vi "Vision Shooter Auto Target.vi"(11 "navX Device":T1={"Interface"={"Protocol"=enum."SERIAL", "Update Rate (4Hz-60Hz)"=4, "navX Open TypeDef"=variant}, "Notify Packet"=refnum, "Loop VI Refnum"=refnum, "Ready to Close Occurrence Refnum"=refnum} {"Interface"."Update Rate (4Hz-60Hz)" min=4 max=60 step=1}) -> ()   [LabVIEW 2015]
uses:
  NavX/navX Library v2/TypeDefs/Z900_navX_DeviceTypeDef.ctl
  NavX/navX Library v2/TypeDefs/Z900_navX_ProtocolTypeDef.ctl
  NavX/navX Library v2/TypeDefs/Z900_navX_NotifyPacketTypeDef.ctl
  NavX/navX Library v2/TypeDefs/Z900_navX_ActionTypeDef.ctl
  Team Code/Robot Global Data.vi
  <vilib>/Rock Robotics/Network Tables/NT Write Number.vi
  NavX/navX Library v2/navX Library v2.lvlib
panel:
  in  "Vertical Linear Relationship":dbl
  out "VisionVertical":cluster{"VisionGyroTarget":dbl, dbl, dbl}(graph)
  out "VisionStateDistance":enum16{"Disabled", "Enable", "Suspended", "PID"}(ring)
  in  "VeriticalOffset":dbl=0.033
  in  "X Gain":dbl=80.0
  in  "minimumVisionValue":dbl=0.45
  out "VisionHorizontal":cluster{"VisionGyroTarget":dbl, dbl, dbl}(graph)
  out "VisionStateAngle":enum16{"Disabled", "Enable", "Suspended", "PID"}(ring)
  in  "HorizontalOffset":dbl=0.066
  # "More positive = counter clockwise\nMore negative = clockwise"
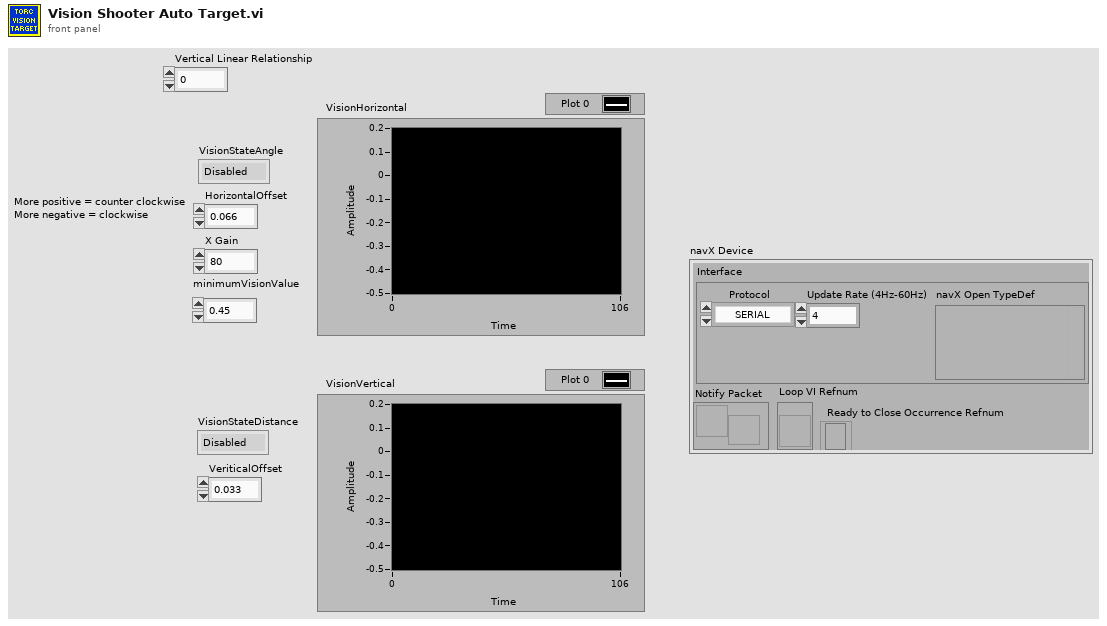
[diagram p1: front panel]
types:
  T1 = typedef "navX Library v2.lvlib/Z900_navX_DeviceTypeDef.ctl" = cluster{"Interface":cluster{"Protocol":T2, "Update Rate (4Hz-60Hz)":u8, "navX Open TypeDef":variant}, "Notify Packet":refnum<notifier>, "Loop VI Refnum":refnum<vi>, "Ready to Close Occurrence Refnum":refnum<k4>}
  T2 = typedef "navX Library v2.lvlib/Z900_navX_ProtocolTypeDef.ctl" = enum16{"SERIAL", "I2C", "SPI"}
  T3 = cluster{"Yaw":dbl, "Roll":dbl, "Pitch":dbl, "Heading":dbl, "Fused Heading":dbl}
  T4 = cluster{"Distance (ft)":dbl, "Center":cluster{dbl, dbl}, "Normalized Rect":cluster{"Numeric":dbl, "Numeric 2":dbl, "Numeric 3":dbl, "Numeric 5":dbl}}[]
  T5 = cluster{"Detected Targets[0]":cluster{"Distance (ft)":dbl, "Center":cluster{dbl, dbl}, "Normalized Rect":cluster{"Numeric":dbl, "Numeric 2":dbl, "Numeric 3":dbl, "Numeric 5":dbl}}, "Detected Targets[1]":cluster{"Distance (ft)":dbl, "Center":cluster{dbl, dbl}, "Normalized Rect":cluster{"Numeric":dbl, "Numeric 2":dbl, "Numeric 3":dbl, "Numeric 5":dbl}}, "Detected Targets[2]":cluster{"Distance (ft)":dbl, "Center":cluster{dbl, dbl}, "Normalized Rect":cluster{"Numeric":dbl, "Numeric 2":dbl, "Numeric 3":dbl, "Numeric 5":dbl}}, "Detected Targets[3]":cluster{"Distance (ft)":dbl, "Center":cluster{dbl, dbl}, "Normalized Rect":cluster{"Numeric":dbl, "Numeric 2":dbl, "Numeric 3":dbl, "Numeric 5":dbl}}, "Detected Targets[4]":cluster{"Distance (ft)":dbl, "Center":cluster{dbl, dbl}, "Normalized Rect":cluster{"Numeric":dbl, "Numeric 2":dbl, "Numeric 3":dbl, "Numeric 5":dbl}}, "Detected Targets[5]":cluster{"Distance (ft)":dbl, "Center":cluster{dbl, dbl}, "Normalized Rect":cluster{"Numeric":dbl, "Numeric 2":dbl, "Numeric 3":dbl, "Numeric 5":dbl}}, "Detected Targets[6]":cluster{"Distance (ft)":dbl, "Center":cluster{dbl, dbl}, "Normalized Rect":cluster{"Numeric":dbl, "Numeric 2":dbl, "Numeric 3":dbl, "Numeric 5":dbl}}, "Detected Targets[7]":cluster{"Distance (ft)":dbl, "Center":cluster{dbl, dbl}, "Normalized Rect":cluster{"Numeric":dbl, "Numeric 2":dbl, "Numeric 3":dbl, "Numeric 5":dbl}}, "Detected Targets[8]":cluster{"Distance (ft)":dbl, "Center":cluster{dbl, dbl}, "Normalized Rect":cluster{"Numeric":dbl, "Numeric 2":dbl, "Numeric 3":dbl, "Numeric 5":dbl}}}
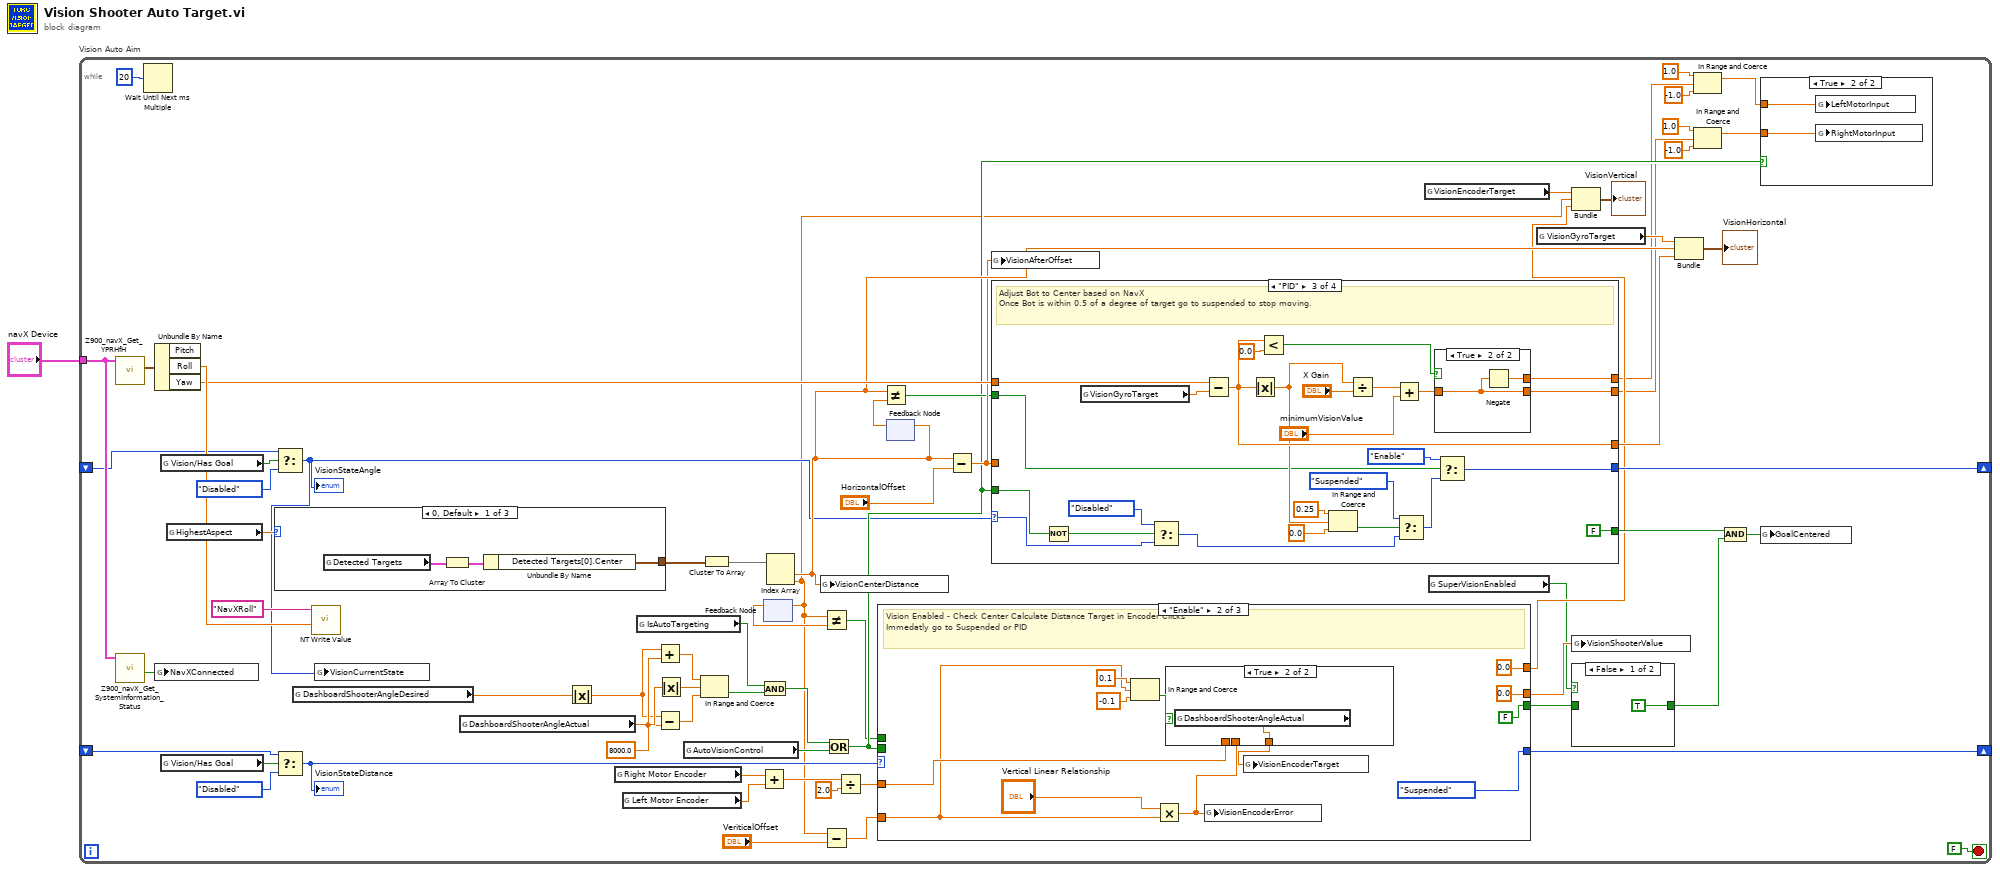
[diagram p0: block diagram]
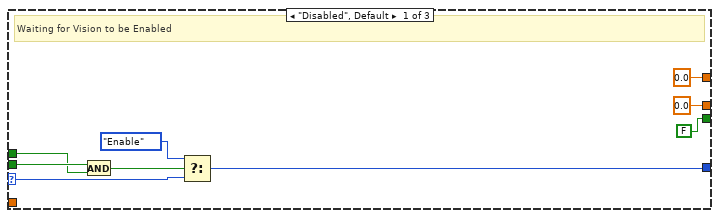
[diagram p3: hidden frame]
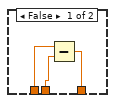
[diagram p4: hidden frame]
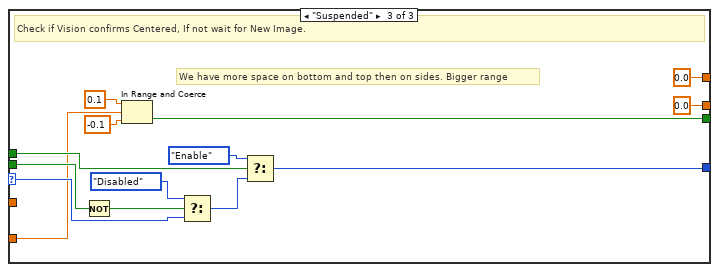
[diagram p5: hidden frame]
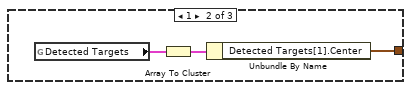
[diagram p6: hidden frame]
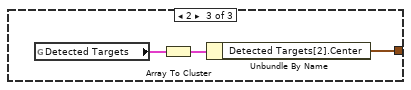
[diagram p7: hidden frame]
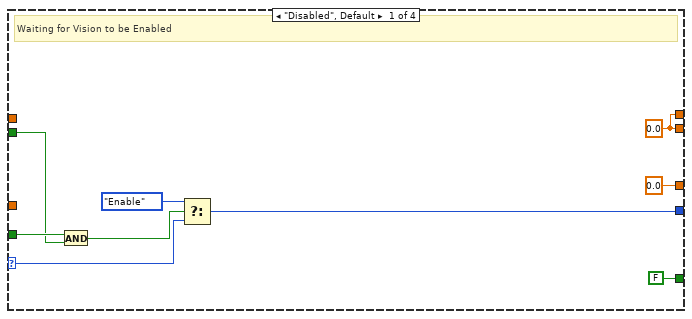
[diagram p9: hidden frame]
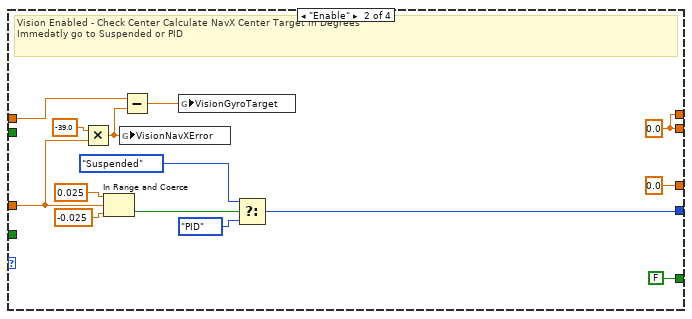
[diagram p10: hidden frame]
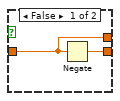
[diagram p11: hidden frame]
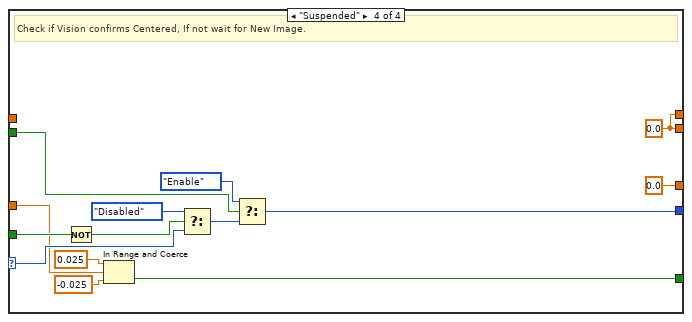
[diagram p12: hidden frame]
diagram:
  n1 = while "Vision Auto Aim" {
    tunnel: "navX Device" -> [w63]
    shift-right: [w66] -> _
    shift-left: _ -> [w49]
    shift-right: [w17] -> _
    shift-left: _ -> [w14]
    stop <- FALSE stop-if-true
    w37 = 8000.0 ("y")
    n2 = call "Z900_navX_Get_YPRHfH.vi"("navX Device"=w63) -> ("YRPHfH"=w67:T3)  [unwired: 7 in, 3 out]
    n3 = call "Z900_navX_Get_SystemInformation_Status.vi"("navX Device"=w63) -> ("Connected"=w50:bool)  [unwired: 7 in, 3 out]
    n4 = Wait Until Next ms Multiple(millisecond multiple=u32 20 ("milliseconds to wait")) -> ()  [unwired: 1 out]
    n5 = Unbundle By Name(w67) -> ("Roll"=w65:dbl, "Yaw"=w44:dbl)  [unwired: 1 out]
    n6 = global write "Robot Global Data.vi" "NavXConnected"(w50) -> ()
    n7 = global read "Robot Global Data.vi" "Vision/Has Goal"() -> (w48:bool)
    n8 = global read "Robot Global Data.vi" "Vision/Has Goal"() -> (w16:bool)
    n9 = global read "Robot Global Data.vi" "HighestAspect"() -> (w46:dbl)
    n10 = case shown="0, Default" w46 {
      tunnel: [w111 w114 w117] -> w53
      frame 0, Default {
        n11 = global read "Robot Global Data.vi" "Detected Targets"() -> (w112:T4)
        n12 = Array To Cluster(array=w112) -> (cluster=w113:T5)
        n13 = Unbundle By Name(w113) -> ("Detected Targets[0].Center"=w111:cluster{dbl, dbl})
      }
      frame 1 {
        n14 = global read "Robot Global Data.vi" "Detected Targets"() -> (w115:T4)
        n15 = Array To Cluster(array=w115) -> (cluster=w116:T5)
        n16 = Unbundle By Name(w116) -> ("Detected Targets[1].Center"=w114:cluster{dbl, dbl})
      }
      frame 2 {
        n17 = global read "Robot Global Data.vi" "Detected Targets"() -> (w118:T4)
        n18 = Array To Cluster(array=w118) -> (cluster=w119:T5)
        n19 = Unbundle By Name(w119) -> ("Detected Targets[2].Center"=w117:cluster{dbl, dbl})
      }
    }
    n20 = Select(t=w49, s=w48, f=enum16{"Disabled", "Enable", "Suspended", "PID"}."Disabled" ("t")) -> (s? t:f=w20:enum16{"Disabled", "Enable", "Suspended", "PID"})
    "VisionStateAngle" <- w20
    n21 = Select(t=w14, s=w16, f=enum16{"Disabled", "Enable", "Suspended", "PID"}."Disabled" ("t")) -> (s? t:f=w13:enum16{"Disabled", "Enable", "Suspended", "PID"})
    "VisionStateDistance" <- w13
    n22 = global read "Robot Global Data.vi" "DashboardShooterAngleDesired"() -> (w39:dbl)
    n23 = call-poly <vilib>:"NT Write Value.vi"("Numeric"=w65, "Name"="NavXRoll") -> ()  [unwired: 9 in, 1 out]
    n24 = global write "Robot Global Data.vi" "VisionCurrentState"(w20) -> ()
    n25 = global read "Robot Global Data.vi" "DashboardShooterAngleActual"() -> (w42:dbl)
    n26 = Absolute Value(x=w39) -> (abs(x)=w36:dbl)
    n27 = global read "Robot Global Data.vi" "Right Motor Encoder"() -> (w25:dbl)
    n28 = global read "Robot Global Data.vi" "Left Motor Encoder"() -> (w24:dbl)
    n29 = global read "Robot Global Data.vi" "IsAutoTargeting"() -> (w35:bool)
    n30 = Add(x=w36, y=w37) -> (x+y=w41:dbl)
    n31 = Subtract(x=w36, y=w37) -> (x-y=w40:dbl)
    n32 = Absolute Value(x=w42) -> (abs(x)=w38:dbl)
    n33 = global read "Robot Global Data.vi" "AutoVisionControl"() -> (w51:bool)
    n34 = In Range and Coerce(upper limit=w41, x=w38, lower limit=w40) -> (In Range?=w34:bool)  [unwired: 1 out]
    n35 = Cluster To Array(cluster=w53) -> (array=w12:dbl[])
    n36 = Add(x=w25, y=w24) -> (x+y=w23:dbl)
    n37 = And(x=w35, y=w34) -> (x .and. y?=w33:bool)
    n38 = feedback #1() -> (w29:dbl)  [unwired: 1 in]
    n39 = Index Array(array=w12) -> (element #1=w43:dbl, element #2=w10:dbl)  [unwired: 2 in]
    n40 = feedback-in #1(w10) -> ()
    n41 = global write "Robot Global Data.vi" "VisionCenterDistance"(w43) -> ()
    n42 = Not Equal?(x=w10, y=w29) -> (x != y?=w26:bool)
    n43 = Subtract(x=w10, y="VeriticalOffset") -> (x-y=w27:dbl)
    n44 = Or(x=w33, y=w51) -> (x .or. y?=w30:bool)
    n45 = Divide(x=w23, y=2.0) -> (x/y=w21:dbl)
    n46 = case shown="\"Enable\"" w13 {
      selector: w13 -> [w80 _ w100]
      tunnel: w30 -> [w76 _ w102]
      tunnel: [w78 enum16{"Disabled", "Enable", "Suspended", "PID"}."Suspended" ("t") w101] -> w17
      tunnel: w21 -> [_ w85 _]
      tunnel: [FALSE FALSE w98] -> w3
      tunnel: w27 -> [_ w81 w97]
      tunnel: [0.0 0.0 ("LeftMotorOutput") 0.0 ("LeftMotorOutput")] -> w5
      tunnel: [0.0 0.0 0.0] -> w8
      tunnel: w26 -> [w72 _ w99]
      frame "Disabled", Default {
        # "Waiting for Vision to be Enabled"
        n47 = And(x=w76, y=w72) -> (x .and. y?=w73:bool)
        n48 = Select(t=enum16{"Disabled", "Enable", "Suspended", "PID"}."Enable", s=w73, f=w80) -> (s? t:f=w78:enum16{"Disabled", "Enable", "Suspended", "PID"})
      }
      frame "Enable" {
        # "Vision Enabled - Check Center Calculate Distance Target in Encoder Clicks\nImmedatly go to Suspended or PID"
        n49 = In Range and Coerce(upper limit=0.1, x=w81, lower limit=-0.1) -> (In Range?=w82:bool)  [unwired: 1 out]
        n50 = Multiply(x="Vertical Linear Relationship", y=w81) -> (x*y=w84:dbl)
        n51 = case shown="True" w82 {
          tunnel: w85 -> [w94 _]
          tunnel: w84 -> [w95 _]
          tunnel: [w93 w96] -> w83
          frame False {
            n52 = Subtract(x=w94, y=w95) -> (x-y=w93:dbl)
          }
          frame True {
            n53 = global read "Robot Global Data.vi" "DashboardShooterAngleActual"() -> (w96:dbl)
          }
        }
        n54 = global write "Robot Global Data.vi" "VisionEncoderError"(w84) -> ()
        n55 = global write "Robot Global Data.vi" "VisionEncoderTarget"(w83) -> ()
      }
      frame "Suspended" {
        # "We have more space on bottom and top then on sides. Bigger range"
        # "Check if Vision confirms Centered, If not wait for New Image."
        n56 = Not(x=w102) -> (.not. x?=w103:bool)
        n57 = In Range and Coerce(upper limit=0.1, x=w97, lower limit=-0.1) -> (In Range?=w98:bool)  [unwired: 1 out]
        n58 = Select(t=enum16{"Disabled", "Enable", "Suspended", "PID"}."Disabled" ("f"), s=w103, f=w100) -> (s? t:f=w105:enum16{"Disabled", "Enable", "Suspended", "PID"})
        n59 = Select(t=enum16{"Disabled", "Enable", "Suspended", "PID"}."Enable" ("f"), s=w99, f=w105) -> (s? t:f=w101:enum16{"Disabled", "Enable", "Suspended", "PID"})
      }
    }
    n60 = feedback-in #2(w43) -> ()
    n61 = feedback #2() -> (w52:dbl)  [unwired: 1 in]
    n62 = Not Equal?(x=w43, y=w52) -> (x != y?=w31:bool)
    n63 = Subtract(x=w43, y="HorizontalOffset") -> (x-y=w32:dbl)
    n64 = global write "Robot Global Data.vi" "VisionAfterOffset"(w32) -> ()
    n65 = case shown="\"PID\"" w20 {
      selector: w20 -> [w130 _ w146 w178]
      tunnel: w30 -> [w126 _ w149 w180]
      tunnel: [w128 w142 w151 w179] -> w66
      tunnel: w44 -> [_ w135 w158 _]
      tunnel: [FALSE FALSE FALSE w176] -> w19
      tunnel: w32 -> [_ w131 _ w175]
      tunnel: [w125 w138 w160 w188] -> w7
      tunnel: [w125 w138 w161 w188] -> w6
      tunnel: [0.0 0.0 w157 0.0] -> w55
      tunnel: w31 -> [w122 _ w145 w177]
      frame "Disabled", Default {
        w125 = 0.0
        # "Waiting for Vision to be Enabled"
        n66 = And(x=w126, y=w122) -> (x .and. y?=w123:bool)
        n67 = Select(t=enum16{"Disabled", "Enable", "Suspended", "PID"}."Enable", s=w123, f=w130) -> (s? t:f=w128:enum16{"Disabled", "Enable", "Suspended", "PID"})
      }
      frame "Enable" {
        w138 = 0.0 ("LeftMotorOutput")
        # "Vision Enabled - Check Center Calculate NavX Center Target in Degrees\nImmedatly go to Suspended or PID"
        n68 = Multiply(x=-39.0, y=w131) -> (x*y=w134:dbl)
        n69 = In Range and Coerce(upper limit=0.025, x=w131, lower limit=-0.025) -> (In Range?=w133:bool)  [unwired: 1 out]
        n70 = global write "Robot Global Data.vi" "VisionNavXError"(w134) -> ()
        n71 = Subtract(x=w135, y=w134) -> (x-y=w137:dbl)
        n72 = global write "Robot Global Data.vi" "VisionGyroTarget"(w137) -> ()
        n73 = Select(t=enum16{"Disabled", "Enable", "Suspended", "PID"}."Suspended", s=w133, f=enum16{"Disabled", "Enable", "Suspended", "PID"}."PID" ("t")) -> (s? t:f=w142:enum16{"Disabled", "Enable", "Suspended", "PID"})
      }
      frame "PID" {
        # "Adjust Bot to Center based on NavX\nOnce Bot is within 0.5 of a degree of target go to suspended to stop moving."
        n74 = Not(x=w149) -> (.not. x?=w148:bool)
        n75 = global read "Robot Global Data.vi" "VisionGyroTarget"() -> (w167:dbl)
        n76 = Select(t=enum16{"Disabled", "Enable", "Suspended", "PID"}."Disabled", s=w148, f=w146) -> (s? t:f=w147:enum16{"Disabled", "Enable", "Suspended", "PID"})
        n77 = Subtract(x=w158, y=w167) -> (x-y=w157:dbl)
        n78 = Absolute Value(x=w157) -> (abs(x)=w155:dbl)
        n79 = Less?(x=w157, y=0.0) -> (x < y?=w163:bool)
        n80 = In Range and Coerce(upper limit=0.25, x=w155, lower limit=0.0) -> (In Range?=w170:bool)  [unwired: 1 out]
        n81 = Divide(x=w155, y="X Gain") -> (x/y=w165:dbl)
        n82 = Add(x=w165, y="minimumVisionValue") -> (x+y=w162:dbl)
        n83 = Select(t=enum16{"Disabled", "Enable", "Suspended", "PID"}."Suspended", s=w170, f=w147) -> (s? t:f=w152:enum16{"Disabled", "Enable", "Suspended", "PID"})
        n84 = case shown="True" w163 {
          tunnel: w162 -> [w172 w173]
          tunnel: [w171 w173] -> w161
          tunnel: [w172 w174] -> w160
          frame False {
            n85 = Negate(x=w172) -> (-x=w171:dbl)
          }
          frame True {
            n86 = Negate(x=w173) -> (-x=w174:dbl)
          }
        }
        n87 = Select(t=enum16{"Disabled", "Enable", "Suspended", "PID"}."Enable", s=w145, f=w152) -> (s? t:f=w151:enum16{"Disabled", "Enable", "Suspended", "PID"})
      }
      frame "Suspended" {
        w188 = 0.0 ("LeftMotorOutput")
        # "Check if Vision confirms Centered, If not wait for New Image."
        n88 = Not(x=w180) -> (.not. x?=w181:bool)
        n89 = In Range and Coerce(upper limit=0.025, x=w175, lower limit=-0.025) -> (In Range?=w176:bool)  [unwired: 1 out]
        n90 = Select(t=enum16{"Disabled", "Enable", "Suspended", "PID"}."Disabled" ("f"), s=w181, f=w178) -> (s? t:f=w183:enum16{"Disabled", "Enable", "Suspended", "PID"})
        n91 = Select(t=enum16{"Disabled", "Enable", "Suspended", "PID"}."Enable" ("f"), s=w177, f=w183) -> (s? t:f=w179:enum16{"Disabled", "Enable", "Suspended", "PID"})
      }
    }
    n92 = global read "Robot Global Data.vi" "VisionEncoderTarget"() -> (w11:dbl)
    n93 = global read "Robot Global Data.vi" "SuperVisionEnabled"() -> (w4:bool)
    n94 = global read "Robot Global Data.vi" "VisionGyroTarget"() -> (w56:dbl)
    n95 = Bundle("VisionEncoderTarget"=w11, w10, w8) -> (→"VisionVertical":cluster{"VisionEncoderTarget":dbl, dbl, dbl})  [unwired: 1 in]
    n96 = global write "Robot Global Data.vi" "VisionShooterValue"(w5) -> ()
    n97 = case shown="False" w4 {
      tunnel: [TRUE w71] -> w2
      tunnel: w3 -> [_ w71]
      frame False {
      }
      frame True {
      }
    }
    n98 = Bundle("VisionGyroTarget"=w56, w43, w55) -> (→"VisionHorizontal":cluster{"VisionGyroTarget":dbl, dbl, dbl})  [unwired: 1 in]
    n99 = In Range and Coerce(upper limit=1.0, x=w7, lower limit=-1.0) -> (coerced(x)=w58:dbl)  [unwired: 1 out]
    n100 = In Range and Coerce(upper limit=1.0, x=w6, lower limit=-1.0) -> (coerced(x)=w57:dbl)  [unwired: 1 out]
    n101 = And(x=w19, y=w2) -> (x .and. y?=w18:bool)
    n102 = case shown="True" w30 {
      tunnel: w57 -> [_ w120]
      tunnel: w58 -> [_ w121]
      frame False {
      }
      frame True {
        n103 = global write "Robot Global Data.vi" "LeftMotorInput"(w121) -> ()
        n104 = global write "Robot Global Data.vi" "RightMotorInput"(w120) -> ()
      }
    }
    n105 = global write "Robot Global Data.vi" "GoalCentered"(w18) -> ()
  }
